vi "create_switch_devices.vi"(8 "error in (no error)":errorcluster) -> (0 "error out":errorcluster)   [LabVIEW 2015]
doc: "reads settings for each switch in \"switches.ini\" and creates objects for each switch. those objects are stored in a global variable. The global variable stores any object no matter what type"
uses:
  Classes/PrepLineObject/PrepLineObject.lvclass
  global variables.vi
  <vilib>/Utility/config.llb/Read Key (String).vi
  <vilib>/Utility/config.llb/Read Key (I32).vi
  <vilib>/Utility/config.llb/Read Key (Boolean).vi
  <vilib>/Utility/config.llb/Read Key (U32).vi
  Classes/StatusLog/StatusLog.lvclass
  <vilib>/Utility/config.llb/NI_LVConfig.lvlib
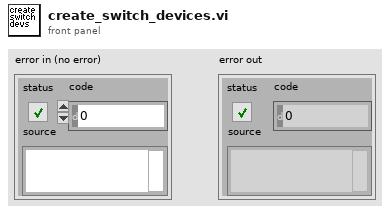
[diagram p1: front panel]
types:
  T1 = typedef "NI_LVConfig.lvlib/Config Data RefNum.ctl" = refnum<k1>
  T2 = typedef "Semaphore RefNum" = refnum<k1>
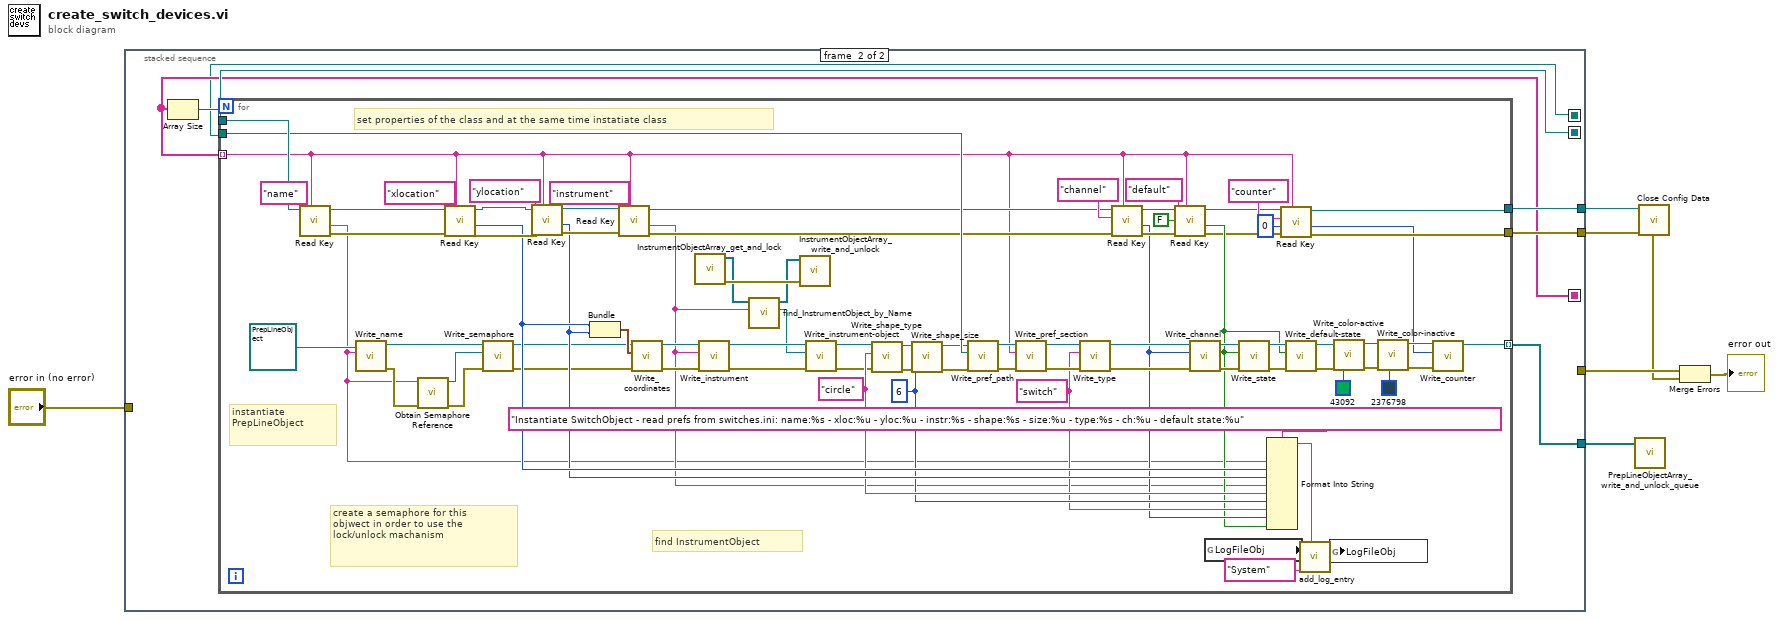
[diagram p0: block diagram]
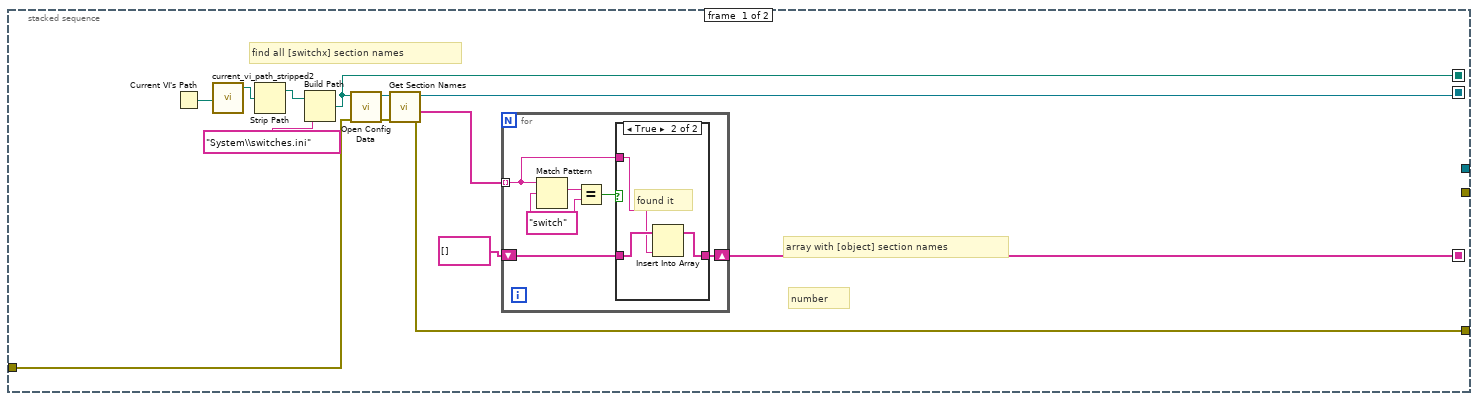
[diagram p2: hidden frame]
diagram:
  n1 = stacked-sequence {
    seq-local: [w16 _] -> [_ w37]
    seq-local: [w12 _] -> [_ w33]
    seq-local: [w11 _] -> [_ w32]
    tunnel: "error in (no error)" -> [w17 _]
    tunnel: [w15 _] -> w6
    tunnel: [_ w36] -> w4
    tunnel: [_ w35] -> w3
    tunnel: [_ w31] -> w1
    frame #0 {
      # "number"
      # "array with [object] section names"
      # "find all [switchx] section names"
      n2 = Current VI's Path() -> (path=w10:path)
      n3 = call "current_vi_path_stripped2.vi"("current VI Path"=w10) -> ("current VI Path stripped out"=w9:path)  [unwired: 3 in, 1 out]
      n4 = Strip Path(path=w9) -> (stripped path=w8:path)  [unwired: 1 out]
      n5 = Build Path(base path=w8, name or relative path="System\\switches.ini") -> (appended path=w11:path)
      n6 = call <vilib>:"Open Config Data.vi"("error in (no error)"=w17, "configuration file path"=w11) -> ("error out"=w18:errorcluster, "refnum"=w19:T1)  [unwired: 7 in, 1 out]
      n7 = call <vilib>:"Get Section Names.vi"("error in (no error)"=w18, "refnum"=w19) -> ("error out"=w15:errorcluster, "section names"=w14:string[], "refnum out"=w16:T1)  [unwired: 7 in]
      n8 = for {
        tunnel: w14 -> [w23] mode=indexing
        shift-right: [w21] -> w12
        shift-left: string[] [] ("section names") -> [w22]
        w25 = "switch" ("regular expression")
        n9 = Match Pattern(string=w23, regular expression=w25) -> (match substring=w26:string)  [unwired: 1 in, 3 out]
        n10 = Equal?(x=w26, y=w25) -> (x = y?=w24:bool)
        n11 = case shown="True" w24 {
          tunnel: w23 -> [_ w29]
          tunnel: [w27 w28] -> w21
          tunnel: w22 -> [w27 w30]
          frame False {
            # "no match"
          }
          frame True {
            # "found it"
            n12 = Insert Into Array(array=w30, new element=w29) -> (w28:string[])  [unwired: 1 in]
          }
        }
      }
    }
    frame #1 {
      n13 = Array Size(array=w33) -> (size(s)=w34:i32)
      n14 = for {
        N: w34 -> [_]
        tunnel: w37 -> [w119]
        tunnel: [w44] -> w36
        tunnel: [w43] -> w35
        tunnel: w33 -> [w47] mode=indexing
        tunnel: w32 -> [w103]
        tunnel: [w40] -> w31 mode=indexing
        w73 = "switch" ("type")
        w74 = i8 6 ("shape type")
        w75 = "circle" ("shape type")
        # "create a semaphore for this\nobjwect in order to use the\nlock/unlock machanism"
        # "find InstrumentObject"
        # "instantiate\nPrepLineObject"
        # "set properties of the class and at the same time instatiate class"
        n15 = call-poly <vilib>:"Read Key.vi"("section"=w47, "key"="name", "refnum"=w119) -> ("error out"=w111:errorcluster, "value"=w54:string, "refnum out"=w114:T1)  [unwired: 5 in, 1 out]
        n16 = call-dynamic "Write_name.vi"("name"=w54, "PrepLinePictureObjects in"=refnum<class "PrepLineObject.lvclass"> refnum ("PrepLineObject.lvclass")) -> ("error out"=w56:errorcluster, "PrepLinePictureObjects out"=w59:refnum<class "PrepLineObject.lvclass">)  [unwired: 8 in]
        n17 = call <vilib>:"Obtain Semaphore Reference.vi"("error in (no error)"=w56, "name (unnamed)"=w54) -> ("error out"=w55:errorcluster, "semaphore"=w53:T2)  [unwired: 3 in, 1 out]
        n18 = call-poly <vilib>:"Read Key.vi"("section"=w47, "error in (no error)"=w111, "key"="xlocation", "refnum"=w114) -> ("error out"=w110:errorcluster, "value"=w77:i32, "refnum out"=w113:T1)  [unwired: 4 in, 1 out]
        n19 = call-dynamic "Write_semaphore.vi"("error in (no error)"=w55, "semaphore"=w53, "PrepLineObject in"=w59) -> ("error out"=w57:errorcluster, "PrepLineObject out"=w58:refnum<class "PrepLineObject.lvclass">)  [unwired: 7 in]
        n20 = call-poly <vilib>:"Read Key.vi"("section"=w47, "error in (no error)"=w110, "key"="ylocation", "refnum"=w113) -> ("error out"=w109:errorcluster, "value"=w76:i32, "refnum out"=w112:T1)  [unwired: 4 in, 1 out]
        n21 = Bundle("value"=w77, "value"=w76) -> (w108:cluster{"value":i32, "value":i32})  [unwired: 1 in]
        n22 = call-poly <vilib>:"Read Key.vi"("section"=w47, "error in (no error)"=w109, "key"="instrument", "refnum"=w112) -> ("error out"=w87:errorcluster, "value"=w60:string, "refnum out"=w88:T1)  [unwired: 4 in, 1 out]
        n23 = call-dynamic "Write_coordinates.vi"("error in (no error)"=w57, "Coords"=w108, "PrepLinePictureObjects in"=w58) -> ("error out"=w106:errorcluster, "PrepLinePictureObjects out"=w107:refnum<class "PrepLineObject.lvclass">)  [unwired: 7 in]
        n24 = call "InstrumentObjectArray_get_and_lock.vi"() -> ("error out"=w52:errorcluster, "InstrumentsObjects"=w51:refnum<class "instrument.lvclass">[])  [unwired: 10 in]
        n25 = call-dynamic "Write_instrument.vi"("error in (no error)"=w106, "instrument name"=w60, "PrepLinePictureObjects in"=w107) -> ("error out"=w61:errorcluster, "PrepLinePictureObjects out"=w62:refnum<class "PrepLineObject.lvclass">)  [unwired: 7 in]
        n26 = call "find_InstrumentObject_by_Name.vi"("Instrument Name"=w60, "InstrumentObjects"=w51) -> ("found InstrObject out"=w49:refnum<class "instrument.lvclass">, "InstrumentObjects out"=w50:refnum<class "instrument.lvclass">[])  [unwired: 6 in, 2 out]
        n27 = call "InstrumentObjectArray_write_and_unlock.vi"("error in (no error)"=w52, "InstrumentObjects"=w50) -> ()  [unwired: 9 in, 1 out]
        n28 = call-dynamic "Write_instrument-object.vi"("error in (no error)"=w61, "instrument.lvclass"=w49, "PrepLineObject in"=w62) -> ("error out"=w63:errorcluster, "PrepLineObject out"=w64:refnum<class "PrepLineObject.lvclass">)  [unwired: 7 in]
        n29 = call-dynamic "Write_shape_type.vi"("error in (no error)"=w63, "shape type"=w75, "PrepLinePictureObjects in"=w64) -> ("error out"=w97:errorcluster, "PrepLinePictureObjects out"=w98:refnum<class "PrepLineObject.lvclass">)  [unwired: 7 in]
        n30 = call-dynamic "Write_shape_size.vi"("error in (no error)"=w97, "shape type"=w74, "PrepLinePictureObjects in"=w98) -> ("error out"=w95:errorcluster, "PrepLinePictureObjects out"=w96:refnum<class "PrepLineObject.lvclass">)  [unwired: 7 in]
        n31 = call-dynamic "Write_pref_path.vi"("error in (no error)"=w95, "pref path"=w103, "PrepLinePictureObjects in"=w96) -> ("error out"=w104:errorcluster, "PrepLinePictureObjects out"=w105:refnum<class "PrepLineObject.lvclass">)  [unwired: 7 in]
        n32 = call-dynamic "Write_pref_section.vi"("error in (no error)"=w104, "pref section"=w47, "PrepLinePictureObjects in"=w105) -> ("error out"=w85:errorcluster, "PrepLinePictureObjects out"=w86:refnum<class "PrepLineObject.lvclass">)  [unwired: 7 in]
        n33 = call-dynamic "Write_type.vi"("error in (no error)"=w85, "device type"=w73, "PrepLinePictureObjects in"=w86) -> ("error out"=w83:errorcluster, "PrepLinePictureObjects out"=w84:refnum<class "PrepLineObject.lvclass">)  [unwired: 7 in]
        n34 = call-poly <vilib>:"Read Key.vi"("section"=w47, "error in (no error)"=w87, "key"="channel", "refnum"=w88) -> ("error out"=w94:errorcluster, "value"=w72:i32, "refnum out"=w93:T1)  [unwired: 4 in, 1 out]
        n35 = call-poly <vilib>:"Read Key.vi"("section"=w47, "error in (no error)"=w94, "default value"=FALSE, "key"="default", "refnum"=w93) -> ("error out"=w45:errorcluster, "value"=w65:bool, "refnum out"=w46:T1)  [unwired: 3 in, 1 out]
        n36 = call-dynamic "Write_channel.vi"("error in (no error)"=w83, "channel"=w72, "PrepLineObject in"=w84) -> ("error out"=w89:errorcluster, "PrepLineObject out"=w90:refnum<class "PrepLineObject.lvclass">)  [unwired: 7 in]
        n37 = global read "global variables.vi" "LogFileObj"() -> (w79:refnum<class "StatusLog.lvclass">)
        n38 = call-dynamic "Write_state.vi"("error in (no error)"=w89, "state"=w65, "PrepLineObject in"=w90) -> ("error out"=w68:errorcluster, "PrepLineObject out"=w69:refnum<class "PrepLineObject.lvclass">)  [unwired: 7 in]
        n39 = Format Into String(format string="Instantiate SwitchObject - read prefs from switches.ini: name:%s - xloc:%u - yloc:%u - instr:%s - shape:%s - size:%u - type:%s - ch:%u - default state:%u", w54, w77, w76, w60, w75, w74, w73, w72, w65) -> (resulting string=w78:string)  [unwired: 2 in, 1 out]
        n40 = call-poly <vilib>:"Read Key.vi"("section"=w47, "error in (no error)"=w45, "default value"=u32 0, "key"="counter", "refnum"=w46) -> ("error out"=w43:errorcluster, "value"=w39:u32, "refnum out"=w44:T1)  [unwired: 3 in, 1 out]
        n41 = call-dynamic "Write_default-state.vi"("error in (no error)"=w68, "default state"=w65, "PrepLineObject in"=w69) -> ("error out"=w66:errorcluster, "PrepLineObject out"=w67:refnum<class "PrepLineObject.lvclass">)  [unwired: 7 in]
        n42 = call-dynamic "add_log_entry.vi"("new entry"=w78, "log identifiers"="System", "StatusLog in"=w79) -> ("StatusLog out"=w80:refnum<class "StatusLog.lvclass">)  [unwired: 5 in, 1 out]
        n43 = global write "global variables.vi" "LogFileObj"(w80) -> ()
        n44 = call-dynamic "Write_color-active.vi"("error in (no error)"=w66, "color active"=u32 43092, "PrepLineObject in"=w67) -> ("error out"=w101:errorcluster, "PrepLineObject out"=w102:refnum<class "PrepLineObject.lvclass">)  [unwired: 7 in]
        n45 = call-dynamic "Write_color-inactive.vi"("error in (no error)"=w101, "color inactive"=u32 2376798, "PrepLineObject in"=w102) -> ("error out"=w41:errorcluster, "PrepLineObject out"=w42:refnum<class "PrepLineObject.lvclass">)  [unwired: 7 in]
        n46 = call-dynamic "Write_counter.vi"("error in (no error)"=w41, "counter"=w39, "PrepLineObject in"=w42) -> ("PrepLineObject out"=w40:refnum<class "PrepLineObject.lvclass">)  [unwired: 7 in, 1 out]
      }
    }
  }
  n47 = call "PrepLineObjectArray_write_and_unlock_queue.vi"("PrepLineObjArray"=w1) -> ()  [unwired: 10 in, 1 out]
  n48 = call <vilib>:"Close Config Data.vi"("error in (no error)"=w3, "refnum"=w4) -> ("error out"=w2:errorcluster)  [unwired: 8 in, 1 out]
  n49 = Merge Errors(w6, w2) -> (→"error out":errorcluster)
